vi "calc_rotate_direction.vi"(1 "control stick":cluster{"roll":i32, "pitch":i32} {"roll" scale=-180.0..180.0; "pitch" scale=-180.0..180.0}, 2 "rotate in":cluster{"pitch":dbl, "roll":dbl, "yaw":dbl} {"pitch" scale=-180.0..180.0; "roll" scale=-180.0..180.0; "yaw" scale=-180.0..180.0}) -> (0 "rotate out":cluster{"pitch":dbl, "roll":dbl, "yaw":dbl} {"pitch" scale=-90.0..90.0; "roll" scale=-90.0..90.0; "yaw" scale=-90.0..90.0})   [LabVIEW 2011]
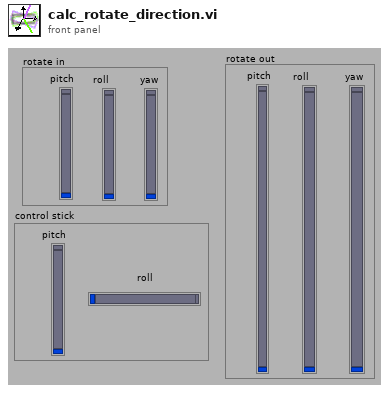
[diagram p1: front panel]
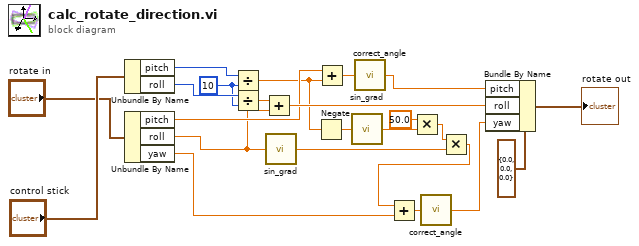
[diagram p0: block diagram]
diagram:
  w10 = 10 ("y")
  n1 = Unbundle By Name("control stick") -> ("pitch"=w15:i32, "roll"=w16:i32)
  n2 = Unbundle By Name("rotate in") -> ("pitch"=w19:dbl, "roll"=w17:dbl, "yaw"=w18:dbl)
  n3 = Divide(x=w15, y=w10) -> (x/y=w12:dbl)
  n4 = Divide(x=w16, y=w10) -> (x/y=w9:dbl)
  n5 = Add(x=w9, y=w17) -> (x+y=w22:dbl)
  n6 = call "sin_grad.vi"("angle out"=w17) -> ("Numeric"=w5:dbl)
  n7 = Negate(x=w12) -> (-x=w11:dbl)
  n8 = Add(x=w19, y=w12) -> (x+y=w3:dbl)
  n9 = call "sin_grad.vi"("angle out"=w11) -> ("Numeric"=w8:dbl)
  n10 = call "correct_angle.vi"("angle in"=w3) -> ("angle out"=w21:dbl)
  n11 = Multiply(x=50.0, y=w8) -> (x*y=w6:dbl)
  n12 = Multiply(x=w6, y=w5) -> (x*y=w13:dbl)
  n13 = Add(x=w13, y=w18) -> (x+y=w4:dbl)
  n14 = call "correct_angle.vi"("angle in"=w4) -> ("angle out"=w23:dbl)
  n15 = Bundle By Name(cluster=cluster{"pitch":dbl, "roll":dbl, "yaw":dbl} {"pitch"=0.0, "roll"=0.0, "yaw"=0.0} ("rotate"), "pitch"=w21, "roll"=w22, "yaw"=w23) -> (→"rotate out":cluster{"pitch":dbl, "roll":dbl, "yaw":dbl})
